vi "RandomNumbers.vi"() -> ()   [LabVIEW 2011]
panel:
  in  "Boolean":bool
  out "Waveform Chart":dbl(graph)
  # "Laborator 7"
  # "Generator de numere aleatoare"
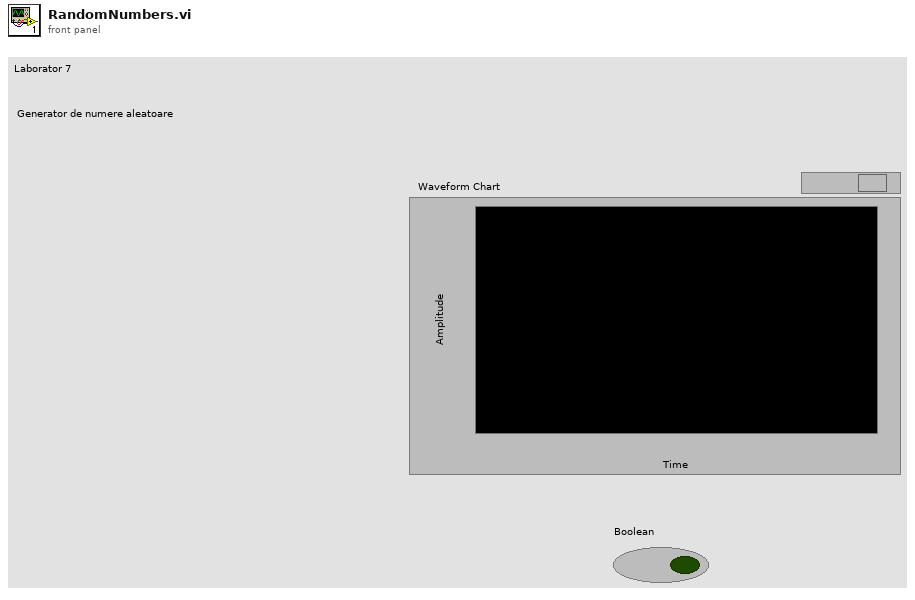
[diagram p1: front panel]
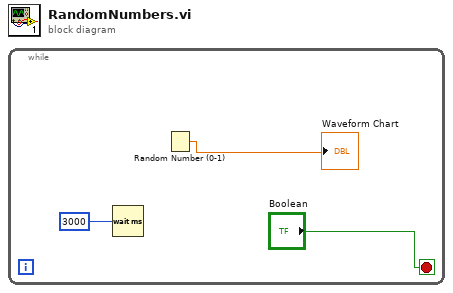
[diagram p0: block diagram]
diagram:
  n1 = while {
    stop <- "Boolean" stop-if-true
    n2 = Wait (ms)(milliseconds to wait=3000) -> ()  [unwired: 1 out]
    n3 = Random Number (0-1)() -> (number: 0 to 1=→"Waveform Chart":dbl)
  }
